vi "TC GUI.vi"() -> ()   [LabVIEW 2016]
uses:
  <vilib>/Utility/file.llb/Write Delimited Spreadsheet (string).vi
  <vilib>/Utility/file.llb/Write Delimited Spreadsheet (DBL).vi
panel:
  in  "base path":path=path "C:/Users/Mark/Desktop/BeadScan"
  out "TC 9Elements":T1 {"Nozzle" format="%#.2g"; "Copper Plate" format="%#.2g"; "Aluminum \nCooling Block" format="%#.2g"; "Bottom\nDowntube" format="%#.2g"; "Top \nDowntube" format="%#.2g"; "Non Optics \nCamera" format="%#.2g"; "Cover Slide Module" format="%#.2g"; "TC #8" format="%#.2g"; "TC #9" format="%#.2g"; "TC #10" format="%#.2g"}
  in  "stop":bool
  out "Waveform Chart":T2(graph)
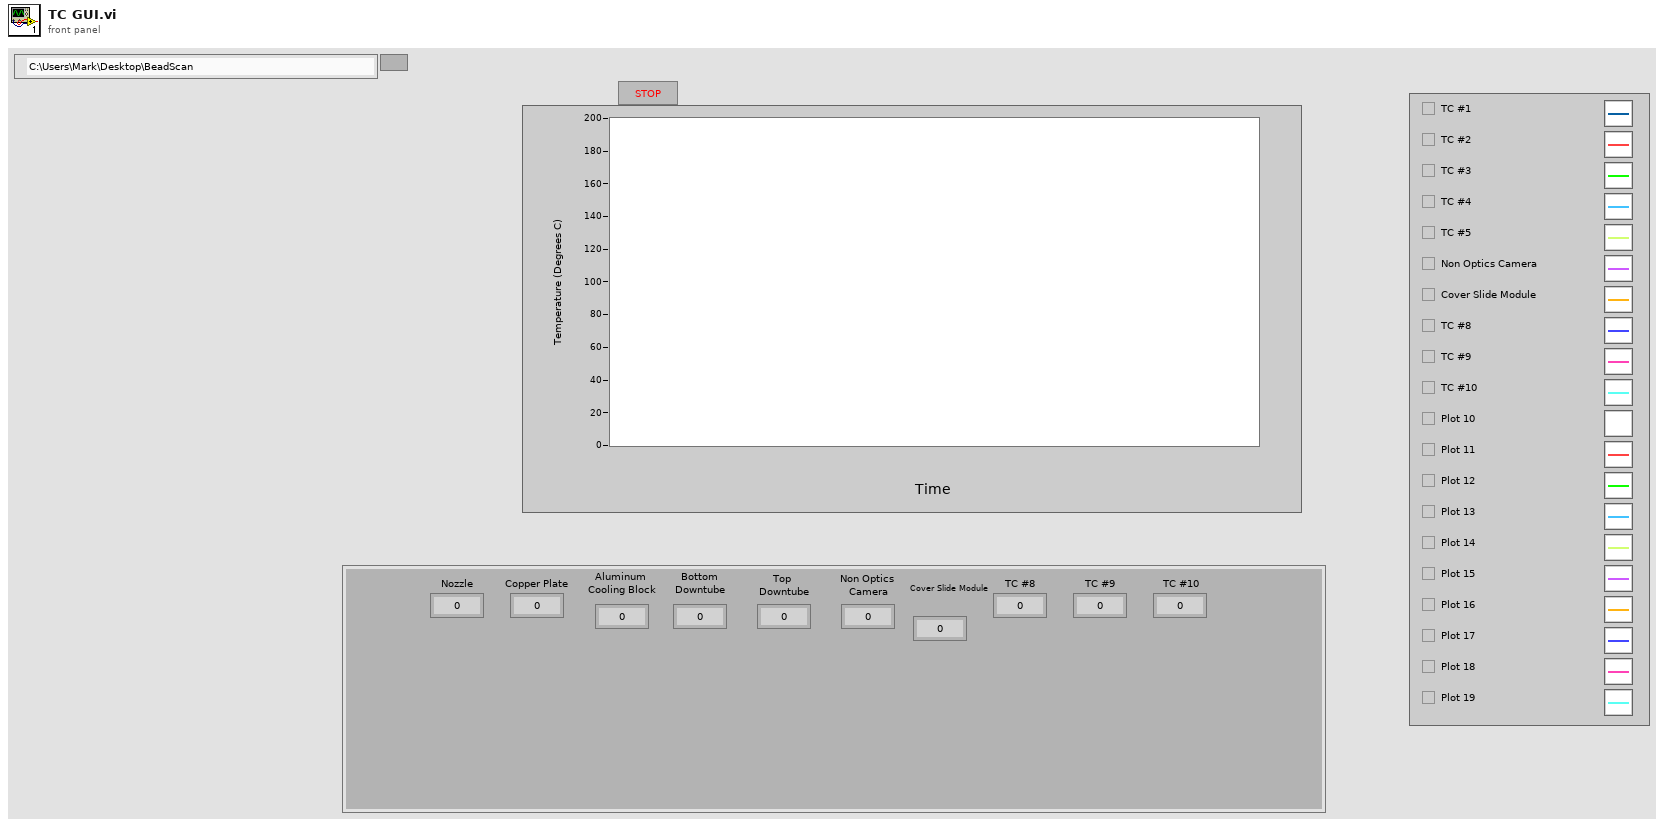
[diagram p1: front panel]
types:
  T1 = cluster{"Nozzle":dbl, "Copper Plate":dbl, "Aluminum \nCooling Block":dbl, "Bottom\nDowntube":dbl, "Top \nDowntube":dbl, "Non Optics \nCamera":dbl, "Cover Slide Module":dbl, "TC #8":dbl, "TC #9":dbl, "TC #10":dbl}
  T2 = cluster{"[0]":dbl, "[1]":dbl, "[2]":dbl, "[3]":dbl, "[4]":dbl, "[5]":dbl, "[6]":dbl, "[7]":dbl, "[8]":dbl, "[9]":dbl}
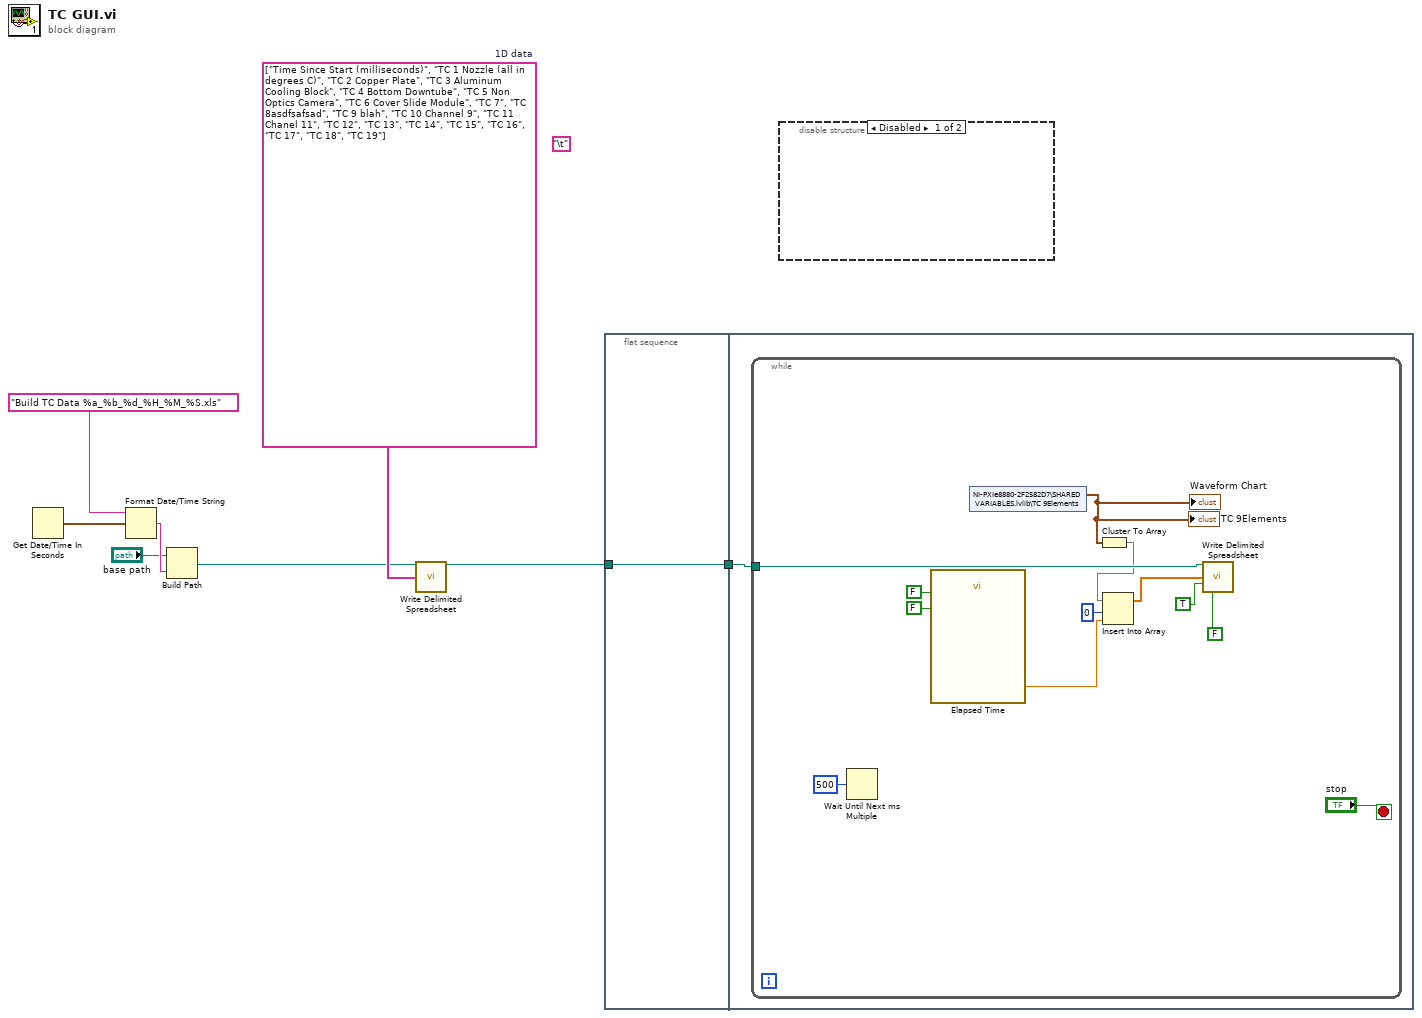
[diagram p0: block diagram]
diagram:
  (unwired) "\t"
  w5 = string[] ["Time Since Start (milliseconds)", "TC 1 Nozzle (all in degrees C)", "TC 2 Copper Plate", "TC 3 Aluminum Cooling Block", "TC 4 Bottom Downtube", "TC 5 Non Optics Camera", "TC 6 Cover Slide Module", "TC 7", "TC 8asdfsafsad", "TC 9 blah", "TC 10 Channel 9", "TC 11 Chanel 11", "TC 12", "TC 13", "TC 14", "TC 15", "TC 16", "TC 17", "TC 18", "TC 19"]  # 1D data
  n1 = Get Date/Time In Seconds() -> (seconds since 1Jan1904=w8:timestamp)
  n2 = Format Date/Time String(time format string (%c)="Build TC Data %a_%b_%d_%H_%M_%S.xls", seconds (now)=w8) -> (date/time string=w6:string)  [unwired: 1 in]
  n3 = Build Path(base path="base path", name or relative path=w6) -> (appended path=w4:path)
  n4 = call-poly <vilib>:"Write Delimited Spreadsheet.vi"("file path (dialog if empty)"=w4, "1D data"=w5) -> ("new file path (Not A Path if cancelled)"=w2:path)  [unwired: 12 in, 1 out]
  n5 = flat-sequence {
    tunnel: w2 -> [w9]
    tunnel: [w9] -> w1
    tunnel: w1 -> [w10]
    frame #0 {
    }
    frame #1 {
      n6 = while {
        tunnel: w10 -> [w20]
        stop <- "stop" stop-if-true
        n7 = Wait Until Next ms Multiple(millisecond multiple=u32 500) -> ()  [unwired: 1 out]
        n8 = call "Elapsed Time"("Reset"=FALSE, "Auto Reset"=FALSE) -> ("Elapsed Time (s)"=w14:dbl)  [unwired: 10 in, 7 out]
        n9 = shared-variable "NI-PXIe8880-2F2582D7\\SHARED VARIABLES.lvlib\\TC 9Elements"() -> (w11:T2)  [unwired: 1 in, 1 out]
        "Waveform Chart" <- w11
        "TC 9Elements" <- w11
        n10 = Cluster To Array(cluster=w11) -> (array=w16:dbl[])
        n11 = Insert Into Array(array=w16, index=0, new element=w14) -> (w15:dbl[])
        n12 = call-poly <vilib>:"Write Delimited Spreadsheet.vi"("file path (dialog if empty)"=w20, "1D data"=w15, "append to file? (new file:F)"=TRUE, "transpose? (no:F)"=FALSE) -> ()  [unwired: 10 in, 2 out]
      }
    }
  }
  n13 = disable-structure shown="Disabled" {
    frame Disabled {
    }
    frame Enabled {
    }
  }
